vi "LVClass_HasoSlopes Save.vi"(0 "HasoSlopes in":refnum<class "HasoSlopes.lvclass">, 5 "path":path, 7 "comments":string, 9 "session":string, 11 "error in (no error)":errorcluster) -> (4 "HasoSlopes out":refnum<class "HasoSlopes.lvclass">, 15 "error out":errorcluster)   [LabVIEW 2020, in "HasoSlopes.lvclass"]
doc: "Save HasoSlopes to a .has file.\n\n--------------------------------------------------------------------------------\n\n<B>HasoSlopesIn </B> : HasoSlopes object.\n<B>HasoSlopesOut </B> : HasoSlopes object.\n<B>has_file_path </B> : Absolute path to the .has file.\n<B>comments </B> : Comments.\n<B>session_name </B> : Session name.\n<B>ErrorIn </B> : Error\n<B>ErrorOut </B> : Error\n\n--------------------------------------------------------------------------------"
uses:
  HasoSlopes.lvclass
  HasoSlopes.lvclass/HasoSlopes.ctl
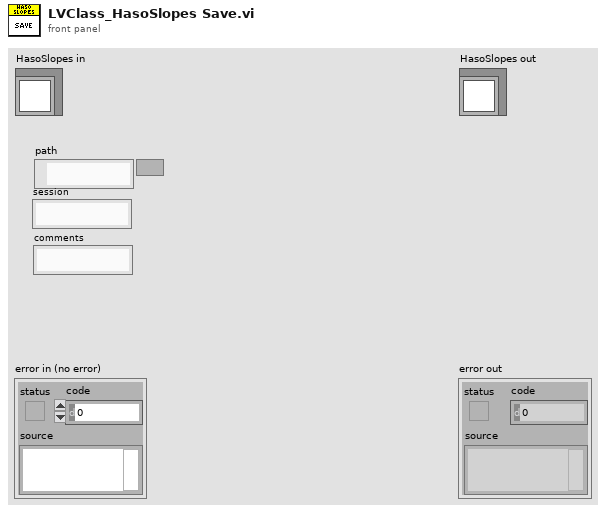
[diagram p1: front panel]
types:
  T1 = enum32{"existing file", "new file", "new or existing file", "existing dir", "new dir", "new or existing dir", "existing file (use LLBs)", "new file (use LLBs)", "new or existing file (use LLBs)", "new or existing file or directory (use LLBs)", "existing dir (use LLBs)", "new dir (use LLBs)", "new or existing dir (use LLBs)", "existing file or dir", "new file or dir", "new or existing file or dir", "existing file or dir (use LLBs)", "new file or dir (use LLBs)", "multi-select", "multi-select (use LLBs)"}
  T2 = typedef "ClassID.ctl" = i64
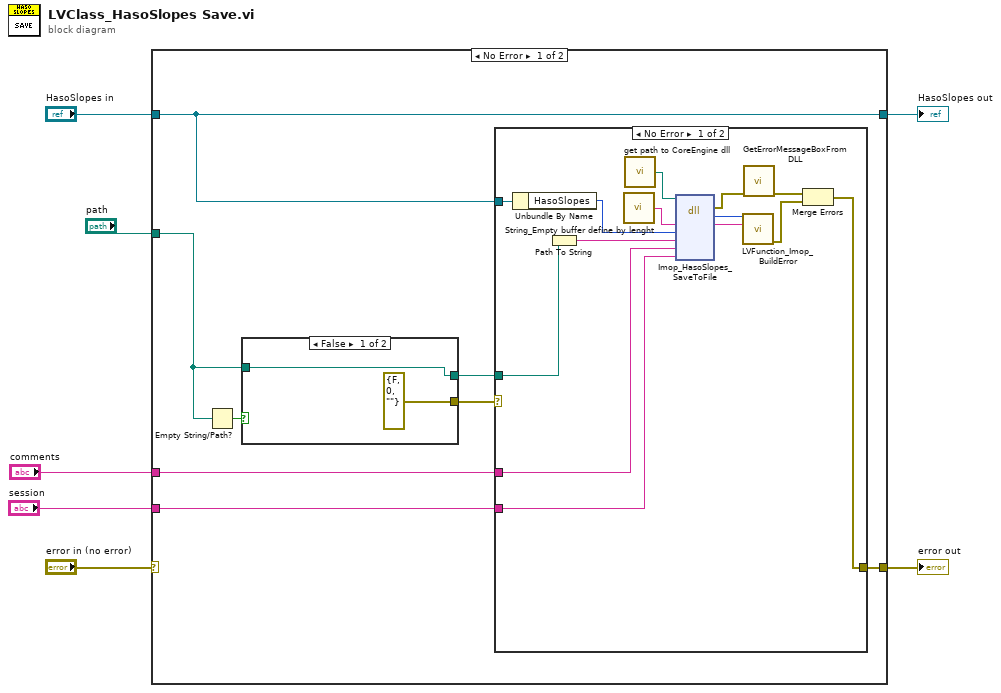
[diagram p0: block diagram]
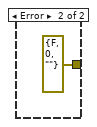
[diagram p2: hidden frame]
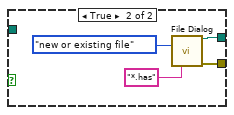
[diagram p3: hidden frame]
diagram:
  n1 = case shown="No Error" "error in (no error)" {
    selector: "error in (no error)" -> [_ w38]
    tunnel: [w14 w38] -> w5
    tunnel: [w15 w37] -> w4
    tunnel: "HasoSlopes in" -> [w15 w37]
    tunnel: "path" -> [w10 _]
    tunnel: "comments" -> [w13 _]
    tunnel: "session" -> [w12 _]
    frame No Error {
      n2 = Empty String/Path?(string/path=w10) -> (empty?=w11:bool)
      n3 = case shown="False" w11 {
        tunnel: [w32 w35] -> w9
        tunnel: w10 -> [w32 _]
        tunnel: [errorcluster {"status"=FALSE, "code"=0, "source"=""} ("error out") w34] -> w8
        frame False {
        }
        frame True {
          n4 = call "File Dialog.vi"("selection mode"=T1."new or existing file", "pattern (all files)"="*.has") -> ("selected path"=w35:path, "error out"=w34:errorcluster)  [unwired: 10 in, 2 out]
        }
      }
      n5 = case shown="No Error" w8 {
        tunnel: w15 -> [w23 _]
        tunnel: [w20 errorcluster {"status"=FALSE, "code"=0, "source"=""} ("error IO")] -> w14
        tunnel: w13 -> [w18 _]
        tunnel: w12 -> [w17 _]
        tunnel: w9 -> [w16 _]
        frame No Error {
          n6 = Unbundle By Name(w23) -> ("HasoSlopes"=w24:T2)
          n7 = Path To String(path=w16) -> (string=w19:string)
          n8 = call "String_Empty buffer define by lenght.vi"() -> ("Empty buffer"=w29:string)  [unwired: 1 in]
          n9 = call "get path to CoreEngine dll.vi"() -> ("path to wavekit library"=w26:path)  [unwired: 14 in, 1 out]
          n10 = dll-call lib="D:/soft/HASO_v3/SVN_trunk/ImOpCoreEngine4_LV2011/DLLs/c_interface_vc100.dll" fn="Imop_HasoSlopes_SaveToFile"(path in=w26, "message"=w29, "HasoSlopes"=w24, "Path"=w19, "comments"=w18, "session"=w17) -> (error out=w25:errorcluster, "return type"=w27:i32, "message"=w28:string)  [unwired: 6 in, 1 out]
          n11 = call "LVFunction_Imop_BuildError.vi"("code"=w27, "String to Prepend to source (\"\")"=w28) -> ("error out"=w21:errorcluster)  [unwired: 13 in]
          n12 = call "GetErrorMessageBoxFromDLL.vi"("error IN"=w25) -> ("error OUT"=w22:errorcluster)  [unwired: 10 in]
          n13 = Merge Errors(w22, w21) -> (w20:errorcluster)
        }
        frame Error {
        }
      }
    }
    frame Error {
    }
  }
  "error out" <- w5
  "HasoSlopes out" <- w4
